vi "DiscoveryService EnumerateServices.vi"(8 "error in":errorcluster, 9 "timeout (ms)":i32=-1, 10 "Request Data":T3, 11 "gRPC ID":T4) -> (0 "error out":errorcluster, 2 "Response Data":T1, 3 "gRPC ID out":T4)   [LabVIEW 2020, in "Discovery_client.lvlib"]
uses:
  Discovery_client.lvlib
  <vilib>/gRPC/LabVIEW gRPC Library/Shared/grpcId.ctl
  RPC Messages/ni_measurements_discovery_v1_EnumerateServicesRequest.ctl
  RPC Messages/ni_measurements_discovery_v1_EnumerateServicesResponse.ctl
  RPC Messages/ni_measurements_discovery_v1_ServiceDescriptor.ctl
  3477ff3c-ac1a-41b2-98e0-1f89dff8fa77.vi
  <vilib>/gRPC/LabVIEW gRPC Library/Shared/TranslateGrpcError.vi
  <vilib>/gRPC/LabVIEW gRPC Library/Shared/Wait On Occurence.vi
  <vilib>/AdvancedString/1D String Array to Delimited String.vi
  <vilib>/gRPC/LabVIEW gRPC Library/Server API/Server/Get Server DLL Path.vi
  <vilib>/gRPC/LabVIEW gRPC Library/grpc-lvsupport-release.lvlib
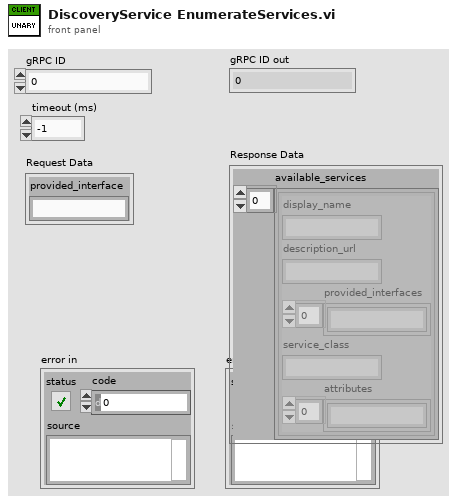
[diagram p1: front panel]
types:
  T1 = typedef "Discovery_client.lvlib/ni_measurements_discovery_v1_EnumerateServicesResponse.ctl" = cluster{"available_services":T2[]}
  T2 = typedef "Discovery_client.lvlib/ni_measurements_discovery_v1_ServiceDescriptor.ctl" = cluster{"display_name":string, "description_url":string, "provided_interfaces":string[], "service_class":string, "attributes":string[]}
  T3 = typedef "Discovery_client.lvlib/ni_measurements_discovery_v1_EnumerateServicesRequest.ctl" = cluster{"provided_interface":string}
  T4 = typedef "grpc-lvsupport-release.lvlib/grpcId.ctl" = u64
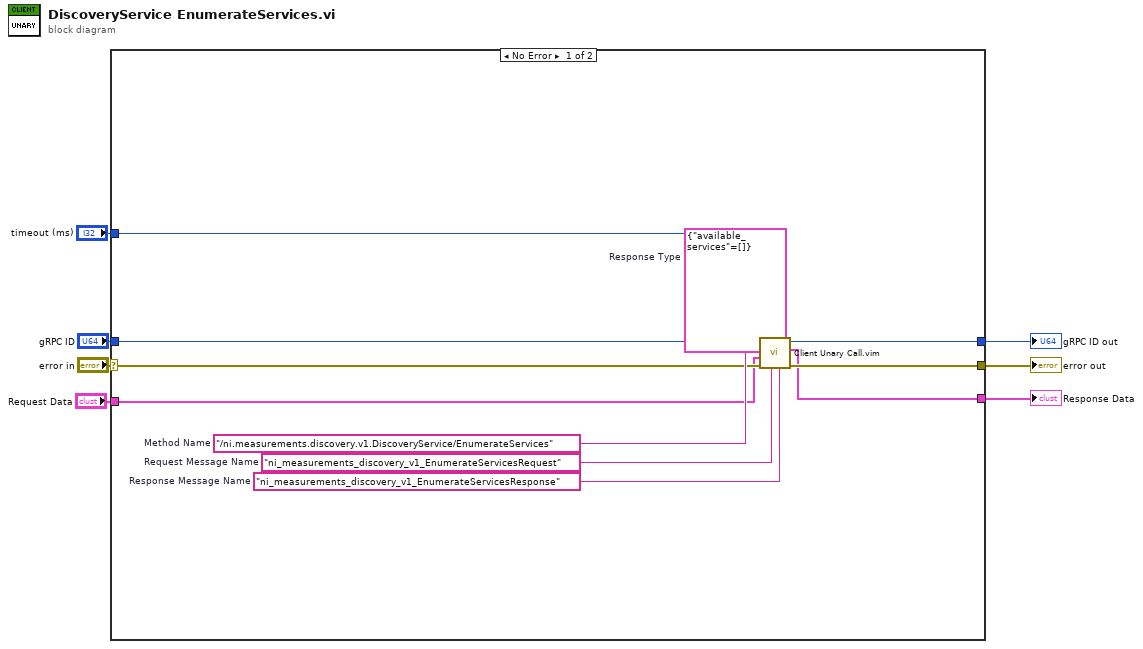
[diagram p0: block diagram]
diagram:
  n1 = case shown="No Error" "error in" {
    selector: "error in" -> [w14 w19]
    tunnel: [w13 w19] -> w6
    tunnel: "gRPC ID" -> [w12 w20]
    tunnel: [w11 w20] -> w4
    tunnel: "Request Data" -> [w10 _]
    tunnel: [w9 _] -> w2
    tunnel: "timeout (ms)" -> [w8 _]
    frame No Error {
      w15 = "ni_measurements_discovery_v1_EnumerateServicesResponse"  # Response Message Name
      w16 = "ni_measurements_discovery_v1_EnumerateServicesRequest"  # Request Message Name
      w17 = T1 {"available_services"=[]}  # Response Type
      w18 = "/ni.measurements.discovery.v1.DiscoveryService/EnumerateServices"  # Method Name
      n2 = call "Client Unary Call.vim"("Response Message Name"=w15, "timeout (ms)"=w8, "Request Message Name"=w16, "Response Type"=w17, "error in"=w14, "Request Data"=w10, "Method Name"=w18, "ClientID in"=w12) -> ("error out"=w13:errorcluster, "Response Data"=w9:T1, "ClientID out"=w11:u64)  [unwired: 1 in]
    }
    frame Error {
    }
  }
  "error out" <- w6
  "gRPC ID out" <- w4
  "Response Data" <- w2
